vi "getDataEndReading.vi"(8 "error in (no error)":errorcluster, 11 "ElectrometerController in":refnum<class "ElectrometerController.lvclass">) -> (0 "error out":errorcluster, 1 "readInitialTime":dbl, 2 "intensities":dbl[](array[numeric]), 3 "ElectrometerController out":refnum<class "ElectrometerController.lvclass">, 4 "temperature":dbl[](array[numeric]), 5 "Units":string[](array[string]))   [LabVIEW 2016, in "ElectrometerController.lvclass"]
uses:
  ElectrometerController.lvclass
  Electrometer/State/ElectrometerState.lvclass
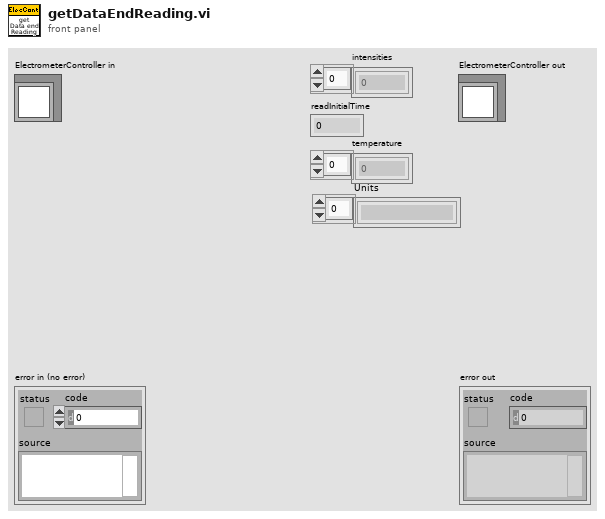
[diagram p1: front panel]
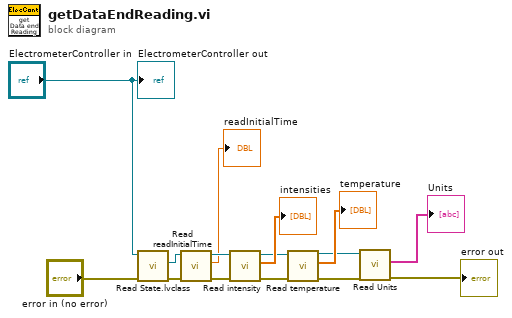
[diagram p0: block diagram]
diagram:
  n1 = call-dynamic "Read State.lvclass.vi"("error in (no error)"="error in (no error)", "ElectrometerController in"="ElectrometerController in") -> ("error out"=w8:errorcluster, "ElectrometerState"=w14:refnum<class "ElectrometerState.lvclass">)  [unwired: 7 in, 1 out]
  n2 = call-dynamic "Read readInitialTime.vi"("error in (no error)"=w8, "State in"=w14) -> ("error out"=w7:errorcluster, "readInitialTime"=→"readInitialTime":dbl, "State out"=w13:refnum<class "ElectrometerState.lvclass">)  [unwired: 7 in]
  n3 = call-dynamic "Read intensity.vi"("error in (no error)"=w7, "State in"=w13) -> ("error out"=w6:errorcluster, "intensity"=→"intensities":dbl[], "State out"=w10:refnum<class "ElectrometerState.lvclass">)  [unwired: 7 in]
  n4 = call-dynamic "Read temperature.vi"("error in (no error)"=w6, "ElectrometerState in"=w10) -> ("error out"=w4:errorcluster, "temperature"=→"temperature":dbl[], "ElectrometerState out"=w2:refnum<class "ElectrometerState.lvclass">)  [unwired: 7 in]
  n5 = call-dynamic "Read Units.vi"("error in (no error)"=w4, "ElectrometerState in"=w2) -> ("error out"=→"error out":errorcluster, "Units"=→"Units":string[])  [unwired: 7 in, 1 out]
  "ElectrometerController out" <- "ElectrometerController in"
